vi "CSV.vi"() -> ()   [LabVIEW 2012]
uses:
  <vilib>/Utility/file.llb/Read From Spreadsheet File (DBL).vi
  <vilib>/Utility/file.llb/Write To Spreadsheet File (DBL).vi
panel:
  in  "Target":path
  in  "Source":path
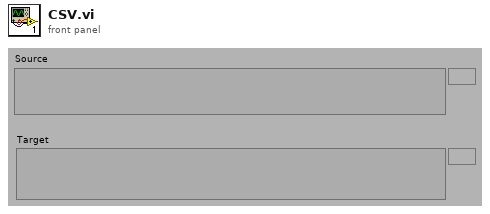
[diagram p1: front panel]
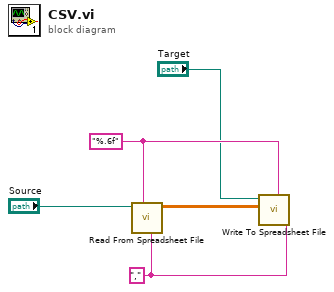
[diagram p0: block diagram]
diagram:
  w2 = "%.6f" ("format (%.3f)")
  w3 = "," ("delimiter (\\t)")
  n1 = call-poly <vilib>:"Read From Spreadsheet File.vi"("delimiter (\\t)"=w3, "format (%.3f)"=w2, "file path (dialog if empty)"="Source") -> ("all rows"=w4:dbl[][])  [unwired: 4 in, 4 out]
  n2 = call-poly <vilib>:"Write To Spreadsheet File.vi"("delimiter (\\t)"=w3, "format (%.3f)"=w2, "2D data"=w4, "file path (dialog if empty)"="Target") -> ()  [unwired: 4 in, 1 out]
